vi "publish -- temperature.vi"(7 "publisher action":T1, 8 "heater IN":dbl=1000.0, 10 "T (K)":dbl=1000.0 format="%#_10f") -> (0 "heater OUT":dbl=1000.0, 2 "T (K) OUT":dbl=1000.0 format="%#_10f")   [LabVIEW 2018]
uses:
  publisher action.ctl
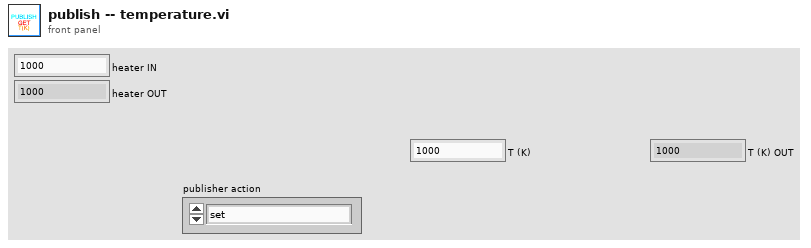
[diagram p1: front panel]
types:
  T1 = typedef "publisher action.ctl" = enum16{"set", "get"}
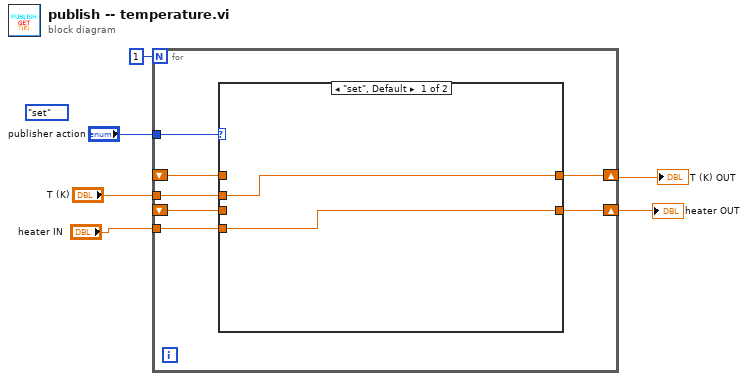
[diagram p0: block diagram]
diagram:
  (unwired) publisher_action."set" ("publisher action")
  n1 = for {
    N: 1 -> [_]
    tunnel: "publisher action" -> [w13]
    tunnel: "T (K)" -> [w11]
    shift-right: [w12] -> w3
    shift-left: _ -> [w10]
    tunnel: "heater IN" -> [w9]
    shift-right: [w8] -> w1
    shift-left: _ -> [w7]
    n2 = case shown="\"set\", Default" w13 {
      tunnel: [w15 w17] -> w12
      tunnel: w11 -> [w15 _]
      tunnel: w10 -> [_ w17]
      tunnel: w9 -> [w14 _]
      tunnel: [w14 w16] -> w8
      tunnel: w7 -> [_ w16]
      frame "set", Default {
      }
      frame "get" {
      }
    }
  }
  "T (K) OUT" <- w3
  "heater OUT" <- w1
